vi "Dst To Dkm.vi"(8 "error in (no error)":errorcluster, 11 "dStations":dbl) -> (0 "error out":errorcluster, 3 "dkm":dbl)   [LabVIEW 2023, in "POSCONV.lvlib"]
doc: "Converts double stations to double kilometres (One station is 100 ft = 0.03048 km)...\n\ndouble DstToDkm(double dStations);"
uses:
  POSCONV.lvlib
  C:/Users/J Gordon/Documents/Rail Tech/TV-HR/02 - Code/Modules/POSCONV/POSCONV.dll
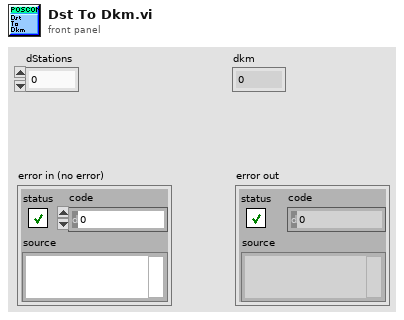
[diagram p1: front panel]
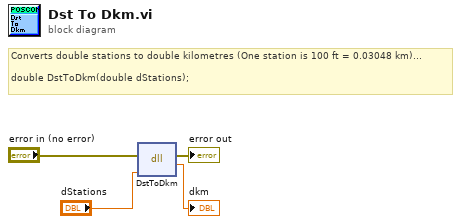
[diagram p0: block diagram]
diagram:
  # "Converts double stations to double kilometres (One station is 100 ft = 0.03048 km)...\n\ndouble DstToDkm(double dStations);"
  n1 = dll-call lib="C:/Users/J Gordon/Documents/Rail Tech/TV-HR/02 - Code/Modules/POSCONV/POSCONV.*" fn="DstToDkm"(error in="error in (no error)", "dStations"="dStations") -> (error out=→"error out":errorcluster, →"dkm":dbl)  [unwired: 3 in, 1 out]
